vi "Oscilloscope.vi"() -> ()   [LabVIEW 2020]
uses:
  <vilib>/DAQmx/read.llb/DAQmx Read (Analog 1D Wfm NChan NSamp).vi
  <vilib>/DAQmx/create/channels.llb/DAQmx Create Channel (AI-Voltage-Basic).vi
  <vilib>/DAQmx/configure/timing.llb/DAQmx Timing (Sample Clock).vi
  <vilib>/DAQmx/miscellaneous.llb/DAQmx Fill In Error Info.vi
panel:
  out "Waveform Graph":waveform(dbl)[](graph)
  in  "Timing Parameters":T1={"Sample Rate (Hz)"=20000, "Samples to Read per Channel"=200} {"Samples to Read per Channel" min=0; "Sample Rate (Hz)" min=0 max=250000 step=1000}
  in  "Channel Parameters":T2={"Device"="Dev1", "Low Channel"=0, "High Channel"=1, "Range"=0.0} {"Range" items=["+/- 10V"=10.0, "+/- 5V"=5.0, "+/- 1V"=1.0, "+/- 0.2V"=0.2]; "High Channel" min=0 max=8; "Low Channel" min=0 max=8}
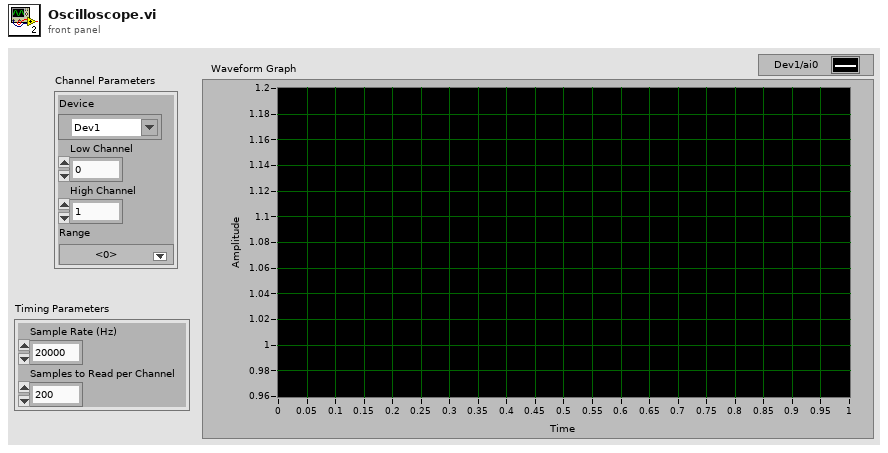
[diagram p1: front panel]
types:
  T1 = cluster{"Sample Rate (Hz)":i32, "Samples to Read per Channel":i32}
  T2 = cluster{"Device":tag, "Low Channel":i32, "High Channel":i32, "Range":dbl}
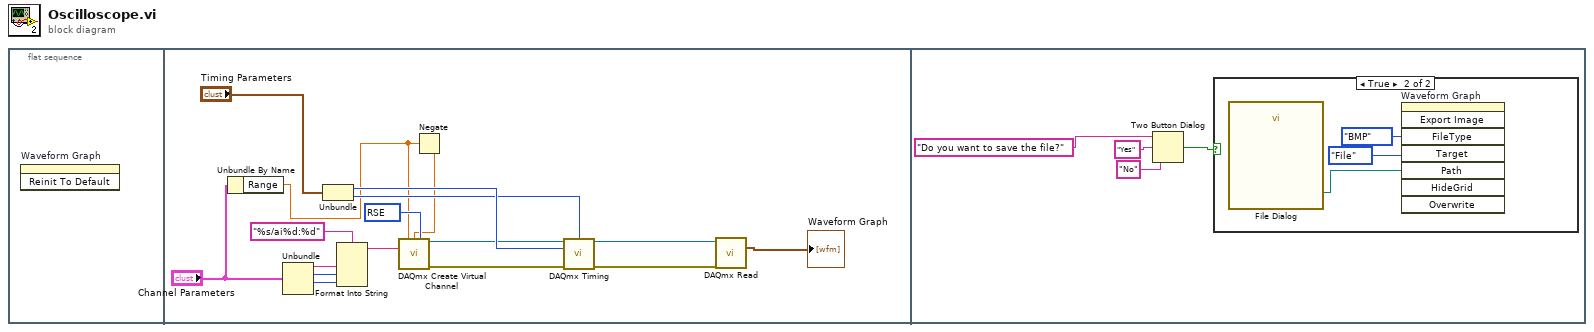
[diagram p0: block diagram]
diagram:
  n1 = flat-sequence {
    frame #0 {
      n2 = invoke on="Waveform Graph" class="WFGraph (strict)" method="Reinit To Default"() -> ()  [unwired: 3 in, 3 out]
    }
    frame #1 {
      w4 = 10083 items=["Default"=-1, "RSE"=10083, "NRSE"=10078, "Differential"=10106, "Pseudodifferential"=12529] ("input terminal configuration")
      n3 = Unbundle By Name("Channel Parameters") -> ("Range"=w2:dbl)
      n4 = Unbundle("Channel Parameters") -> ("Device"=w7:tag, "Low Channel"=w8:i32, "High Channel"=w9:i32)  [unwired: 1 out]
      n5 = Unbundle("Timing Parameters") -> ("Sample Rate (Hz)"=w14:i32, "Samples to Read per Channel"=w5:i32)
      n6 = Format Into String(format string="%s/ai%d:%d" ("initial string"), w7, w8, w9) -> (resulting string=w13:string)  [unwired: 2 in, 1 out]
      n7 = Negate(x=w2) -> (-x=w1:dbl)
      n8 = call-poly <vilib>:"DAQmx Create Virtual Channel.vi"("maximum value"=w2, "minimum value"=w1, "input terminal configuration"=w4, "physical channels"=w13) -> ("task out"=w11:refnum<k21>, "error out"=w12:errorcluster)  [unwired: 10 in]
      n9 = call-poly <vilib>:"DAQmx Timing.vi"("task/channels in"=w11, "samples per channel"=w5, "rate"=w14, "error in"=w12) -> ("task out"=w15:refnum<k21>, "error out"=w16:errorcluster)  [unwired: 10 in]
      n10 = call-poly <vilib>:"DAQmx Read.vi"("task/channels in"=w15, "error in"=w16) -> ("data"=→"Waveform Graph":waveform(dbl)[])  [unwired: 11 in, 2 out]
    }
    frame #2 {
      n11 = Two Button Dialog(message="Do you want to save the file?", 1:"No" ("F button name (\"Cancel\")"), 2:"Yes" ("T button name (\"OK\")")) -> (T button?=w18:bool)
      n12 = case shown="True" w18 {
        frame False {
        }
        frame True {
          n13 = call "File Dialog"() -> ("selected path"=w24:path)  [unwired: 12 in, 3 out]
          n14 = invoke on="Waveform Graph" class="WFGraph (strict)" method="Export Image"("FileType"=enum32{"BMP", "EPS", "EMF", "PICT"}."BMP" ("File Type"), "Target"=enum32{"File", "Clipboard"}."File", "Path"=w24) -> ()  [unwired: 5 in, 8 out]
        }
      }
    }
  }
